vi "Write.ProcessData.vi"(8 "error in":errorcluster, 9 "Offset":i32, 10 "Values":dbl[](array[numeric]), 11 "Write in":refnum<class "Write.lvclass">) -> (0 "error out":errorcluster, 3 "Write out":refnum<class "Write.lvclass">)   [LabVIEW 2024, in "VS Plugin Data Access Engine.lvlib" / "Write.lvclass"]
uses:
  Write.lvclass
  Write.lvclass/Write.ctl
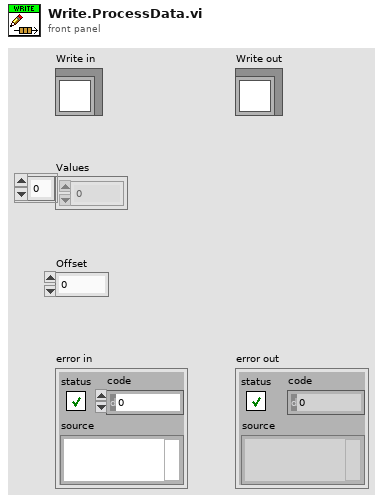
[diagram p1: front panel]
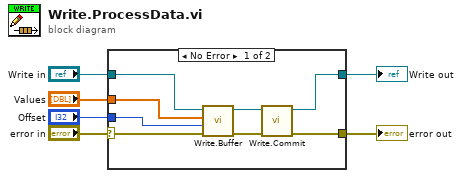
[diagram p0: block diagram]
diagram:
  n1 = case shown="No Error" "error in" {
    selector: "error in" -> [w13 w16]
    tunnel: [w12 w16] -> w5
    tunnel: [w7 w15] -> w1
    tunnel: "Write in" -> [w10 w15]
    tunnel: "Values" -> [w9 _]
    tunnel: "Offset" -> [w8 _]
    frame No Error {
      n2 = call "Write.Buffer.vi"("error in"=w13, "Offset"=w8, "Values"=w9, "Write in"=w10) -> ("error out"=w14:errorcluster, "Write out"=w11:refnum<class "Write.lvclass">)  [unwired: 6 in]
      n3 = call "Write.Commit.vi"("error in"=w14, "Write in"=w11) -> ("error out"=w12:errorcluster, "Write out"=w7:refnum<class "Write.lvclass">)  [unwired: 8 in]
    }
    frame Error {
    }
  }
  "error out" <- w5
  "Write out" <- w1
